vi "Get Time Ref Tab.vi"(11 "Time Ref":T1) -> (3 "TimeRefTab":T2)   [LabVIEW 2018, in "Chassis TimeSync System Explorer.lvlib"]
uses:
  Chassis TimeSync System Explorer.lvlib
  Time Ref Tab.ctl
  Shared/Time Reference.ctl
  Shared/Chassis TimeSync Shared.lvlib
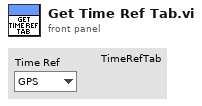
[diagram p1: front panel]
types:
  T1 = typedef "Chassis TimeSync Shared.lvlib/Time Reference.ctl" = enum16{"GPS", "IRIG", "PPS", "1588 Ordinary Clock", "802.1AS", "PXI Chassis Clock", "Free Running (Internal)"}
  T2 = typedef "Chassis TimeSync System Explorer.lvlib/Time Ref Tab.ctl" = enum32{"Empty", "1588", "IRIG", "PPS"}
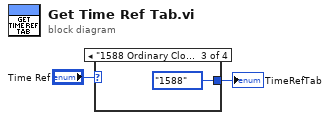
[diagram p0: block diagram]
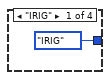
[diagram p2: hidden frame]
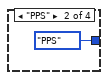
[diagram p3: hidden frame]
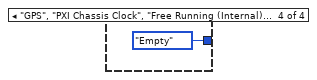
[diagram p4: hidden frame]
diagram:
  n1 = case shown="\"1588 Ordinary Clock\", \"802.1AS\"" "Time Ref" {
    tunnel: [Time_Ref_Tab."IRIG" ("TimeRefTab") Time_Ref_Tab."PPS" ("TimeRefTab") Time_Ref_Tab."1588" ("TimeRefTab") Time_Ref_Tab."Empty" ("TimeRefTab")] -> w2
    frame "IRIG" {
    }
    frame "PPS" {
    }
    frame "1588 Ordinary Clock", "802.1AS" {
    }
    frame "GPS", "PXI Chassis Clock", "Free Running (Internal)" {
    }
  }
  "TimeRefTab" <- w2
